vi "add rows(SubVI).vi"(1 "array in":dbl[][](array[numeric])) -> (0 "array out":dbl[](array[numeric]))   [LabVIEW 2009]
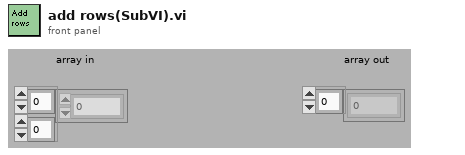
[diagram p1: front panel]
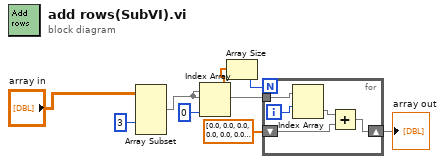
[diagram p0: block diagram]
diagram:
  n1 = Array Subset(array="array in", index (col)=3 ("index")) -> (w6:dbl[][])  [unwired: 3 in]
  n2 = Index Array(array=w6, index (col)=0 ("disabled index (col)")) -> (element=w4:dbl[])  [unwired: 1 in]
  n3 = Array Size(array=w4) -> (size(s)=w3:i32)
  n4 = for {
    N: w3 -> [_]
    tunnel: w6 -> [w13]
    shift-right: [w10] -> w8
    shift-left: dbl[] [0.0, 0.0, 0.0, 0.0, 0.0, 0.0, 0.0, 0.0, 0.0] -> [w9]
    i -> [w12]
    n5 = Index Array(array=w13, index (row)=w12) -> (element=w11:dbl[])  [unwired: 1 in]
    n6 = Add(x=w11, y=w9) -> (x+y=w10:dbl[])
  }
  "array out" <- w8
